vi "Get Monkey Picture.vi"() -> (0 "Monkey":picture)   [LabVIEW 2026, in "TALOS.lvlib"]
uses:
  TALOS.lvlib
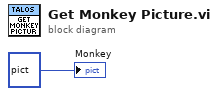
[diagram p0: block diagram]
diagram:
  "Monkey" <- picture bytes[3230] ("Monkey")
